vi "Parse Output Signals.vi"(8 "error in (no error)":errorcluster, 11 "Device Ref in":T3 format="%.0x") -> (0 "error out":errorcluster, 1 "XNET Output Signal Names":refnum<k21>[](array[refnum]), 2 "Input Data Refs":T1[](array[typedef]) {"Data Reference" format="%.0x"}, 3 "Device Ref out":T3=18446744073709551615 format="%.0x", 5 "Input Values":dbl[](array[numeric]))   [LabVIEW 2009, in "NI-XNET Custom Device.lvlib"]
doc: "This VI gets the information from the system explorer and gets a list of signal names."
uses:
  NI-XNET Custom Device.lvlib
  <vilib>/NI VeriStand/Custom Device API/Custom Device Item Ref.ctl
  <vilib>/NI VeriStand/Custom Device API/Block Data Reference.ctl
  <vilib>/NI VeriStand/Custom Device API/Data Reference.ctl
  <vilib>/NI VeriStand/Custom Device API/Custom Device Channel Type.ctl
  <vilib>/NI VeriStand/Custom Device API/Data Access Type.ctl
  <vilib>/NI VeriStand/Custom Device API/Get Item Property (Variant).vi
  <vilib>/NI VeriStand/Custom Device API/Custom Device API.lvlib
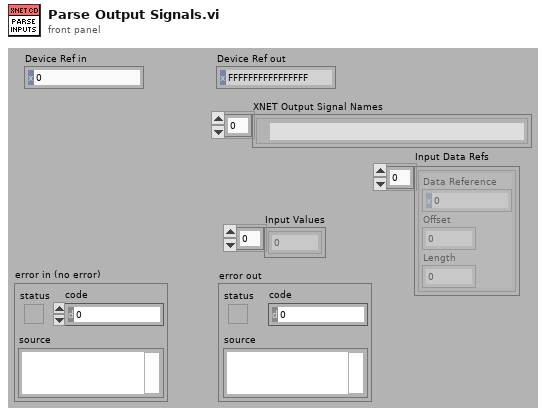
[diagram p1: front panel]
types:
  T1 = typedef "Custom Device API.lvlib/Block Data Reference.ctl" = cluster{"Data Reference":T2, "Offset":i32, "Length":i32}
  T2 = typedef "Custom Device API.lvlib/Data Reference.ctl" = i32
  T3 = typedef "Custom Device API.lvlib/Custom Device Item Ref.ctl" = u64
  T4 = typedef "Custom Device API.lvlib/Data Access Type.ctl" = enum16{"Read", "Write"}
  T5 = typedef "Custom Device API.lvlib/Custom Device Channel Type.ctl" = enum16{"Input", "Output"}
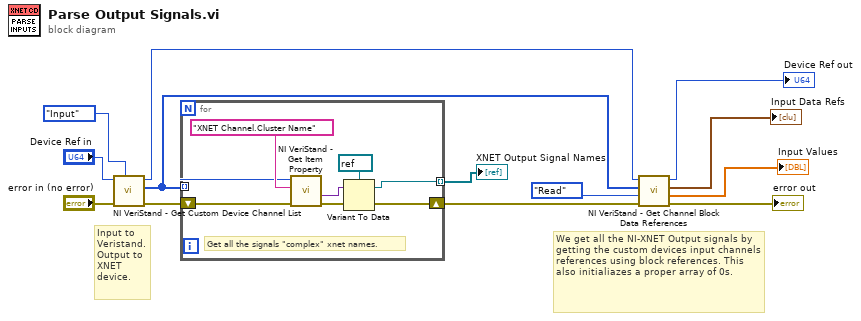
[diagram p0: block diagram]
diagram:
  # "We get all the NI-XNET Output signals by getting the custom devices input channels references using block references. This also initialiazes a proper array of 0s."
  # "Input to Veristand.  Output to XNET device."
  n1 = call <vilib>:"NI VeriStand - Get Custom Device Channel List.vi"("Channel Type"=Custom_Device_Channel_Type."Input", "error in (no error)"="error in (no error)", "Device Ref in"="Device Ref in") -> ("error out"=w13:errorcluster, "Specified Channel Ref List"=w7:T3[], "Device Ref out"=w8:T3)  [unwired: 6 out]
  n2 = for {
    tunnel: w7 -> [w20] mode=indexing
    shift-right: [w16] -> w6
    shift-left: w13 -> [w14]
    tunnel: [w15] -> w9 mode=indexing
    # "Get all the signals \"complex\" xnet names."
    n3 = call-poly <vilib>:"NI VeriStand - Get Item Property.vi"("error in (no error)"=w14, "Property Name"="XNET Channel.Cluster Name", "Item Ref in"=w20) -> ("error out"=w18:errorcluster, "Value"=w17:variant)  [unwired: 5 in, 2 out]
    n4 = Variant To Data(error in=w18, Variant=w17, type=refnum<k21> refnum ("XNET Signal")) -> (error out=w16:errorcluster, data=w15:refnum<k21>)
  }
  "XNET Output Signal Names" <- w9
  n5 = call <vilib>:"NI VeriStand - Get Channel Block Data References.vi"("error in (no error)"=w6, "Access"=Data_Access_Type."Read", "Channel Refs"=w7, "Device Ref in"=w8) -> ("error out"=→"error out":errorcluster, "Values Array"=→"Input Values":dbl[], "Block Data Refs"=→"Input Data Refs":T1[], "Device Ref out"=→"Device Ref out":T3)  [unwired: 4 out]
